vi "Get Image Packed Field.vi"(8 "error in (no error)":errorcluster caption="错误输入（无错误）", 10 "Image Descriptor":T2, 11 "Gif Image 输入":refnum<class "Gif Image.lvclass"> caption="DNL_LabVIEW Object in") -> (0 "error out":errorcluster caption="错误输出", 2 "Image Packed Filed":T1, 3 "Gif Image 输出":refnum<class "Gif Image.lvclass"> caption="DNL_LabVIEW Object out")   [LabVIEW 2012, in "Picture Box Tools.lvlib" / "Gif Image.lvclass"]
uses:
  Gif Image.lvclass
  Control/Image Descriptor.ctl
  Control/Image Packed Field.ctl
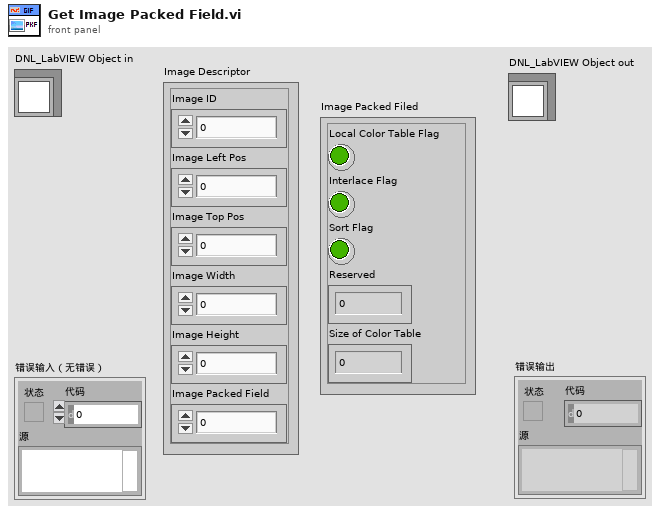
[diagram p1: front panel]
types:
  T1 = typedef "Picture Box Tools.lvlib/Gif Image.lvclass/Image Packed Field.ctl" = cluster{"Local Color Table Flag ":bool, "Interlace Flag":bool, "Sort Flag":bool, "Reserved":u8, "Size of Color Table":u8}
  T2 = typedef "Picture Box Tools.lvlib/Gif Image.lvclass/Image Descriptor.ctl" = cluster{"Image ID":u8, "Image Left Pos":u16, "Image Top Pos":u16, "Image Width":u16, "Image Height":u16, "Image Packed Field":u8}
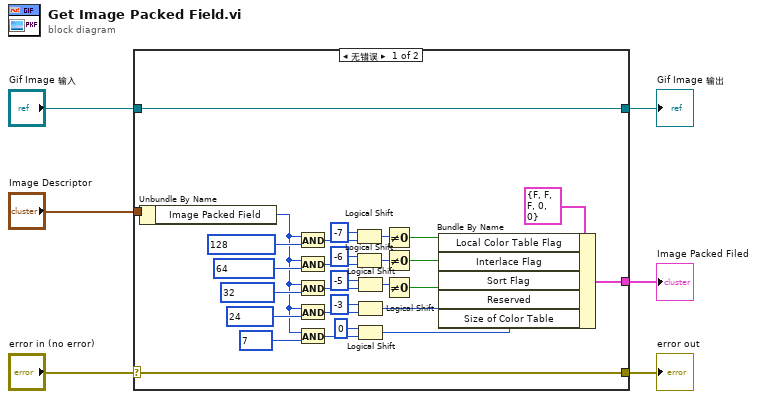
[diagram p0: block diagram]
diagram:
  n1 = case shown="无错误" "error in (no error)" {
    selector: "error in (no error)" -> [w34 w37]
    tunnel: [w34 w37] -> w5
    tunnel: [w35 w36] -> w3
    tunnel: "Gif Image 输入" -> [w35 w36]
    tunnel: "Image Descriptor" -> [w33 _]
    tunnel: [w16 _] -> w1
    frame No Error {
      n2 = Unbundle By Name(w33) -> ("Image Packed Field"=w17:u8)
      n3 = And(x=w17, y=u8 128 ("length (rest)")) -> (x .and. y?=w23:u8)
      n4 = And(x=w17, y=u8 64 ("length (rest)")) -> (x .and. y?=w24:u8)
      n5 = And(x=w17, y=u8 32 ("length (rest)")) -> (x .and. y?=w25:u8)
      n6 = And(x=w17, y=u8 24 ("length (rest)")) -> (x .and. y?=w26:u8)
      n7 = And(x=w17, y=u8 7 ("length (rest)")) -> (x .and. y?=w27:u8)
      n8 = Logical Shift(y=-7 ("length (rest)"), x=w23) -> (x << y=w14:u8)
      n9 = Logical Shift(y=-6 ("length (rest)"), x=w24) -> (x << y=w12:u8)
      n10 = Logical Shift(y=-5 ("length (rest)"), x=w25) -> (x << y=w10:u8)
      n11 = Logical Shift(y=-3 ("length (rest)"), x=w26) -> (x << y=w8:u8)
      n12 = Logical Shift(y=0 ("length (rest)"), x=w27) -> (x << y=w7:u8)
      n13 = Not Equal To 0?(x=w14) -> (x != 0?=w13:bool)
      n14 = Not Equal To 0?(x=w12) -> (x != 0?=w11:bool)
      n15 = Not Equal To 0?(x=w10) -> (x != 0?=w9:bool)
      n16 = Bundle By Name(cluster=T1 {"Local Color Table Flag "=FALSE, "Interlace Flag"=FALSE, "Sort Flag"=FALSE, "Reserved"=0, "Size of Color Table"=0} ("Image Packed Filed"), "Local Color Table Flag"=w13, "Interlace Flag"=w11, "Sort Flag"=w9, "Reserved"=w8, "Size of Color Table"=w7) -> (w16:T1)
    }
    frame Error {
    }
  }
  "error out" <- w5
  "Gif Image 输出" <- w3
  "Image Packed Filed" <- w1
